vi "ImpulseAnalyzer.vi"() -> ()   [LabVIEW 2015]
uses:
  <vilib>/express/express analysis/Spectral/Block/exnSpectralBlock spectral measurements RMS poly.vi
  <vilib>/express/express analysis/Spectral/Block/exnSpectralBlock spectral measurements RMS DDT.vi
  <vilib>/express/express analysis/Spectral/XNode/ExpressSpectralMeasurementsBlockNode.xnode
panel:
  out "FFT":dynamicdata(graph)=[{"t0"=timestamp(0 s since 1904-01-01), "dt"=0.000125, "Y"=array[4000 elements], "attributes"=variant("NI_ChannelName"=variant(string "FFT - (RMS)"))}]
  out "Waveform Graph":dbl[](graph)
  in  "error in":errorcluster
  out "error out":errorcluster
  in  "stop":bool
  in  "Time(s)":dbl=0.2 format="%_1g"
  in  "Rate":dbl=40000.0
  in  "Averages":dbl=10.0
  # "Buffer size of about 170 is where the measurements breakdown"
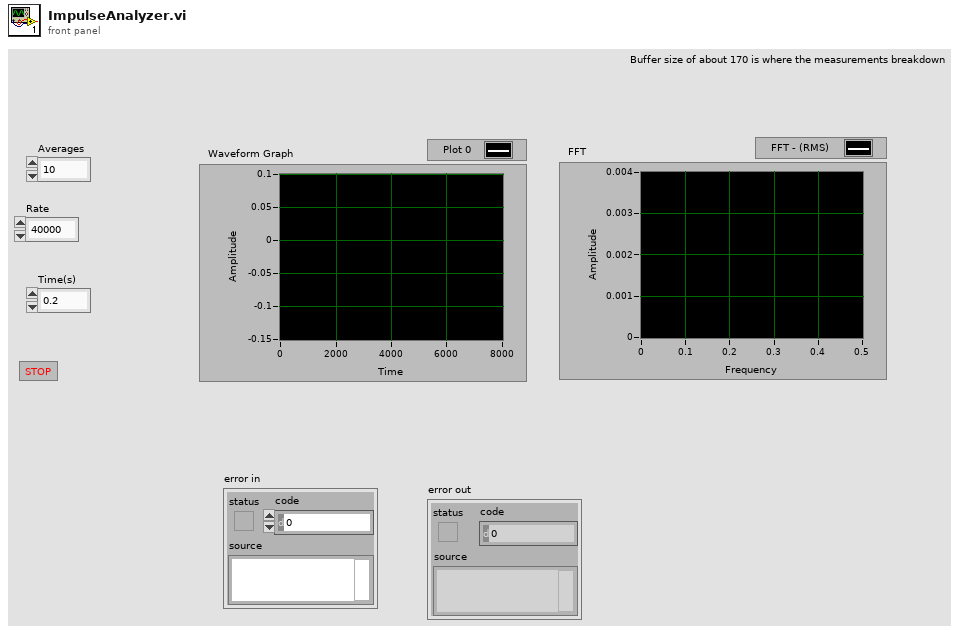
[diagram p1: front panel]
types:
  T1 = cluster{"averaging mode":u16, "weighting mode":u16, "number of averages":u32}
  T2 = cluster{"dB On (F)":bool, "unwrap phase (F)":bool, "convert to degree (F)":bool}
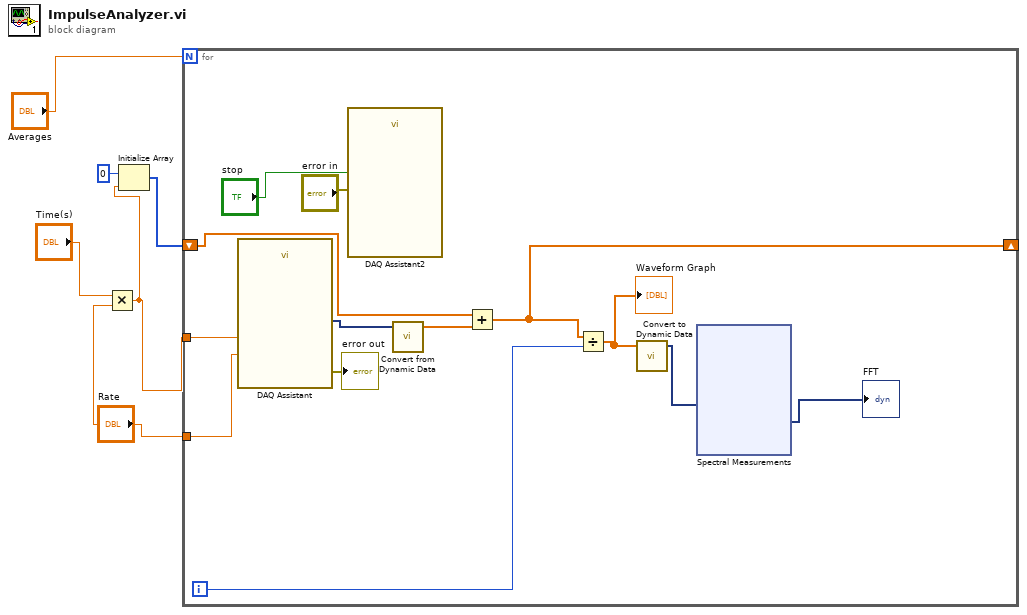
[diagram p0: block diagram]
diagram:
  n1 = Multiply(x="Time(s)", y="Rate") -> (x*y=w1:dbl)
  n2 = Initialize Array(0 ("element"), w1) -> (w3:i32[])
  n3 = for {
    N: "Averages" -> [_]
    shift-right: [w10] -> _
    shift-left: w3 -> [w13]
    tunnel: "Rate" -> [w18]
    tunnel: w1 -> [w7]
    i -> [w12]
    n4 = call "DAQ Assistant"("rate"=w18, "number of samples"=w7) -> ("data"=w16:dynamicdata, "error out"=→"error out":errorcluster)  [unwired: 15 in, 1 out]
    n5 = call "DAQ Assistant2"("error in"="error in", "stop (T)"="stop") -> ()  [unwired: 16 in, 2 out]
    n6 = call "Convert from Dynamic Data"("Dynamic Data Type"=w16) -> ("Array"=w14:dbl[])  [unwired: 3 in]
    n7 = Add(x=w13, y=w14) -> (x+y=w10:dbl[])
    n8 = Divide(x=w10, y=w12) -> (x/y=w11:dbl[])
    "Waveform Graph" <- w11
    n9 = call "Convert to Dynamic Data"("Array"=w11) -> ("Dynamic Data Type"=w9:dynamicdata)  [unwired: 3 in]
    n10 = xnode "Spectral Measurements"("Signals"=w9) -> ("FFT - (RMS)"=→"FFT":dynamicdata)  [unwired: 1 in, 2 out]
  }
